vi "Segments to String.vi"(7 "Separator (dot)":string, 10 "Segments":string[](array[string])) -> (2 "String":string)   [LabVIEW 2020, in "OpenConvert.lvlib"]
uses:
  OpenConvert.lvlib
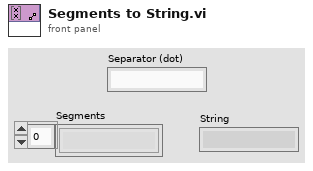
[diagram p1: front panel]
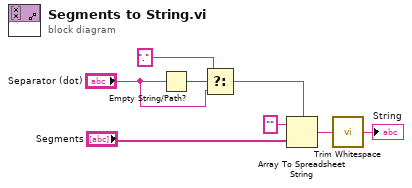
[diagram p0: block diagram]
diagram:
  n1 = Empty String/Path?(string/path="Separator (dot)") -> (empty?=w3:bool)
  n2 = Select(t="." ("delimiter (Tab)"), s=w3, f="Separator (dot)") -> (s? t:f=w6:string)
  n3 = Array To Spreadsheet String(delimiter (Tab)=w6, array="Segments", 3:"" ("format string")) -> (spreadsheet string=w2:string)
  n4 = call <vilib>:"Trim Whitespace.vi"("string"=w2) -> ("trimmed string"=→"String":string)  [unwired: 1 in]
